vi "Init.vi"(8 "error in (no error)":errorcluster, 10 "IConfigure":refnum<class "IConfigure.lvclass">, 11 "Camera Base in":refnum<class "Camera Base.lvclass">) -> (0 "error out":errorcluster, 3 "Camera Base out":refnum<class "Camera Base.lvclass">)   [LabVIEW 2023, in "Camera Base.lvclass"]
uses:
  Camera Base.lvclass
  Camera Base.lvclass/Camera Base.ctl
  Interfaces/IConfigure/IConfigure.lvclass
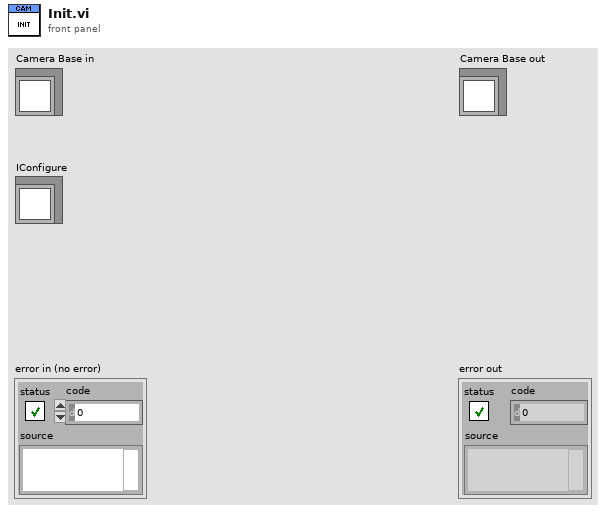
[diagram p1: front panel]
types:
  T1 = typedef "IMAQ Image.ctl" = refnum<image>
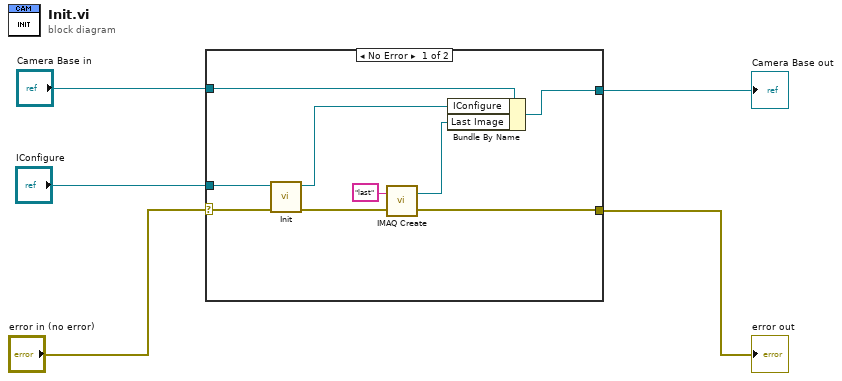
[diagram p0: block diagram]
diagram:
  n1 = case shown="No Error" "error in (no error)" {
    selector: "error in (no error)" -> [w10 w16]
    tunnel: "IConfigure" -> [w14 _]
    tunnel: [w7 w16] -> w4
    tunnel: "Camera Base in" -> [w13 w15]
    tunnel: [w11 w15] -> w2
    frame No Error {
      n2 = call-dynamic "Init.vi"("error in (no error)"=w10, "IConfigure in"=w14) -> ("error out"=w8:errorcluster, "IConfigure out"=w12:refnum<class "IConfigure.lvclass">)  [unwired: 8 in]
      n3 = call "IMAQ Create"("Image Name"="last", "error in (no error)"=w8) -> ("New Image"=w6:T1, "error out"=w7:errorcluster)  [unwired: 3 in]
      n4 = Bundle By Name(cluster=w13, "IConfigure"=w12, "Last Image"=w6) -> (w11:refnum<class "Camera Base.lvclass">)
    }
    frame Error {
    }
  }
  "error out" <- w4
  "Camera Base out" <- w2
